vi "Wrapper 2.vi"(0 "IVI Refnum in":refnum<k15>, 1 "Load SMU":T2 {"Resolution in Digits" items=["3 1/2"=3.5, "4 1/2"=4.5, "5 1/2"=5.5, "6 1/2"=6.5, "7 1/2"=7.5]; "Range (Amps)" format="%.2p"}, 5 "Load SMU 2":refnum<k15>, 7 "Load SMU Channel":string, 9 "Cluster":T1 {"Source Delay (Sec)" format="%.3p"; "Voltage Limit Range" format="%.5p"; "Voltage Limit" format="%.5p"; "Current Level Range" format="%.3p"; "Current Level" format="%.3p"}, 11 "error in (no error)":errorcluster) -> (4 "Name":T3, 15 "error out":errorcluster)   [LabVIEW 2021, in "Different Library t12.lvlib"]
uses:
  Different Library t12.lvlib
  NIDCpower/NIDCPower T12.lvlib
  NIDMM/Meas T12.ctl
  NIDMM/LoadDMM t12.ctl
  NIDCpower/controls/Config.ctl
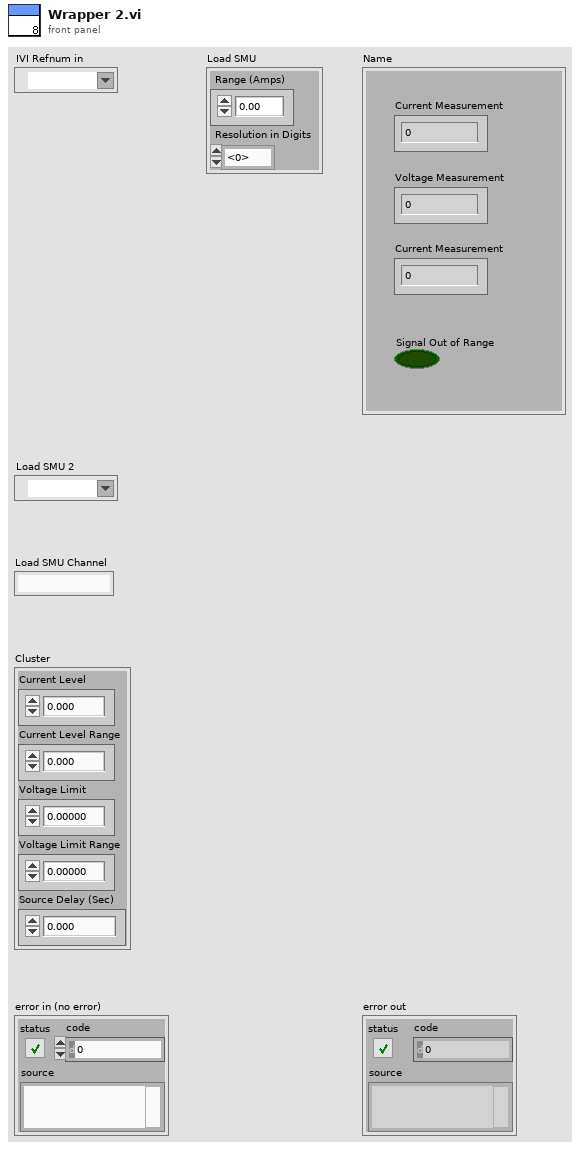
[diagram p1: front panel]
types:
  T1 = typedef "NIDCPower T12.lvlib/Config.ctl" = cluster{"Current Level":dbl, "Current Level Range":dbl, "Voltage Limit":dbl, "Voltage Limit Range":dbl, "Source Delay (Sec)":dbl}
  T2 = typedef "LoadDMM t12.ctl" = cluster{"Range (Amps)":dbl, "Resolution in Digits":dbl}
  T3 = typedef "Meas T12.ctl" = cluster{"Current Measurement":dbl, "Voltage Measurement":dbl, "Signal Out of Range":bool, "Current in DMM":dbl}
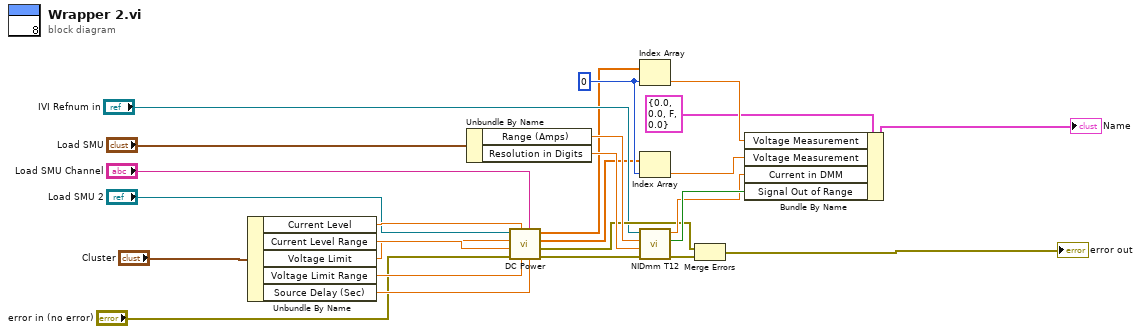
[diagram p0: block diagram]
diagram:
  w3 = 0 ("index")
  n1 = Unbundle By Name("Cluster") -> ("Current Level"=w13:dbl, "Current Level Range"=w15:dbl, "Voltage Limit"=w14:dbl, "Voltage Limit Range"=w16:dbl, "Source Delay (Sec)"=w17:dbl)
  n2 = Unbundle By Name("Load SMU") -> ("Range (Amps)"=w19:dbl, "Resolution in Digits"=w20:dbl)
  n3 = call "DC Power.vi"("Source Delay (Sec)"=w17, "Load SMU Channel"="Load SMU Channel", "Voltage Limit Range"=w16, "Current Level"=w13, "error in (no error)"="error in (no error)", "Current Level Range"=w15, "Voltage Limit"=w14, "IVI Refnum in"="Load SMU 2") -> (0:"error out"=w9:errorcluster, 1:"error out"=w10:errorcluster, "current measurements"=w2:dbl[], "voltage measurements"=w1:dbl[])
  n4 = Index Array(array=w1, index=w3) -> (element=w23:dbl)
  n5 = Index Array(array=w2, index=w3) -> (element=w24:dbl)
  n6 = call "NIDmm T12.vi"("error in (no error)"=w9, "Range (Amps)"=w20, "Resolution in Digits"=w19, "IVI Refnum in"="IVI Refnum in") -> ("error out"=w11:errorcluster, "Over Range?"=w26:bool, "Measurement"=w25:dbl)  [unwired: 5 in]
  n7 = Merge Errors(w10, w11) -> (→"error out":errorcluster)
  n8 = Bundle By Name(cluster=T3 {"Current Measurement"=0.0, "Voltage Measurement"=0.0, "Signal Out of Range"=FALSE, "Current in DMM"=0.0} ("Name"), "Voltage Measurement"=w23, "Voltage Measurement"=w24, "Current in DMM"=w25, "Signal Out of Range"=w26) -> (→"Name":T3)
